vi "AnalyzeGraph.vi"(0 "Grp_Raw":waveform(dbl)[](graph), 5 "start samples/time":dbl caption="시작 샘플/시간" format="%0.2f", 7 "FittingPara":T1={"HorL_Threshold"=0.0, "HorR_Threshold"=0.0, "HorPk Width"=2, "VerL_Threshold"=0.0, "VerR_Threshold"=0.0, "VerPk Width"=2, "TorL_Threshold 3"=0.0, "TorR_Threshold"=0.0, "TorPk Width 3"=2}, 9 "duration":dbl=1.0 caption="지속기간" format="%0.2f") -> (3 "Grp_ExtVel":waveform(dbl)[](graph), 4 "Grp_ExtPos":waveform(dbl)[](graph), 6 "Hor_CycleOut":waveform(dbl)[](array[waveform]), 8 "Table_Out":dbl[][](array[numeric]), 10 "HV_CycleOut":waveform(dbl)(graph), 11 "Basic_Detection":cluster{"period":dbl, "mean":dbl, dbl}, 12 "Ver_CycleOut":waveform(dbl)[](array[waveform]), 13 "SNTable_Out":dbl[][](array[numeric]), 14 "Grph_Dir":bool, 15 "Tor_CycleOut":waveform(dbl)[](array[waveform]))   [LabVIEW 2013]
uses:
  <vilib>/Analysis/baseanly.llb/Mean (DBL).vi
  <vilib>/Waveform/WDTOps.llb/WDT Get Waveform Subset DBL.vi
  <vilib>/Waveform/WDTOps.llb/WDT Waveform Duration DBL.vi
  <vilib>/measure/mascope.llb/Pulse Measurements 1 chan.vi
  <vilib>/addons/Wavelet Analysis/application.llb/WA Multiscale Peak Detection (Waveform).vi
  <vilib>/measure/NI_MAPro.lvlib
  <vilib>/Analysis/NI_AAL_SigProc.lvlib
  <vilib>/Analysis/NI_AALBase.lvlib
  <vilib>/addons/_Advanced Signal Processing/NI_AdvSigProcWA.lvlib
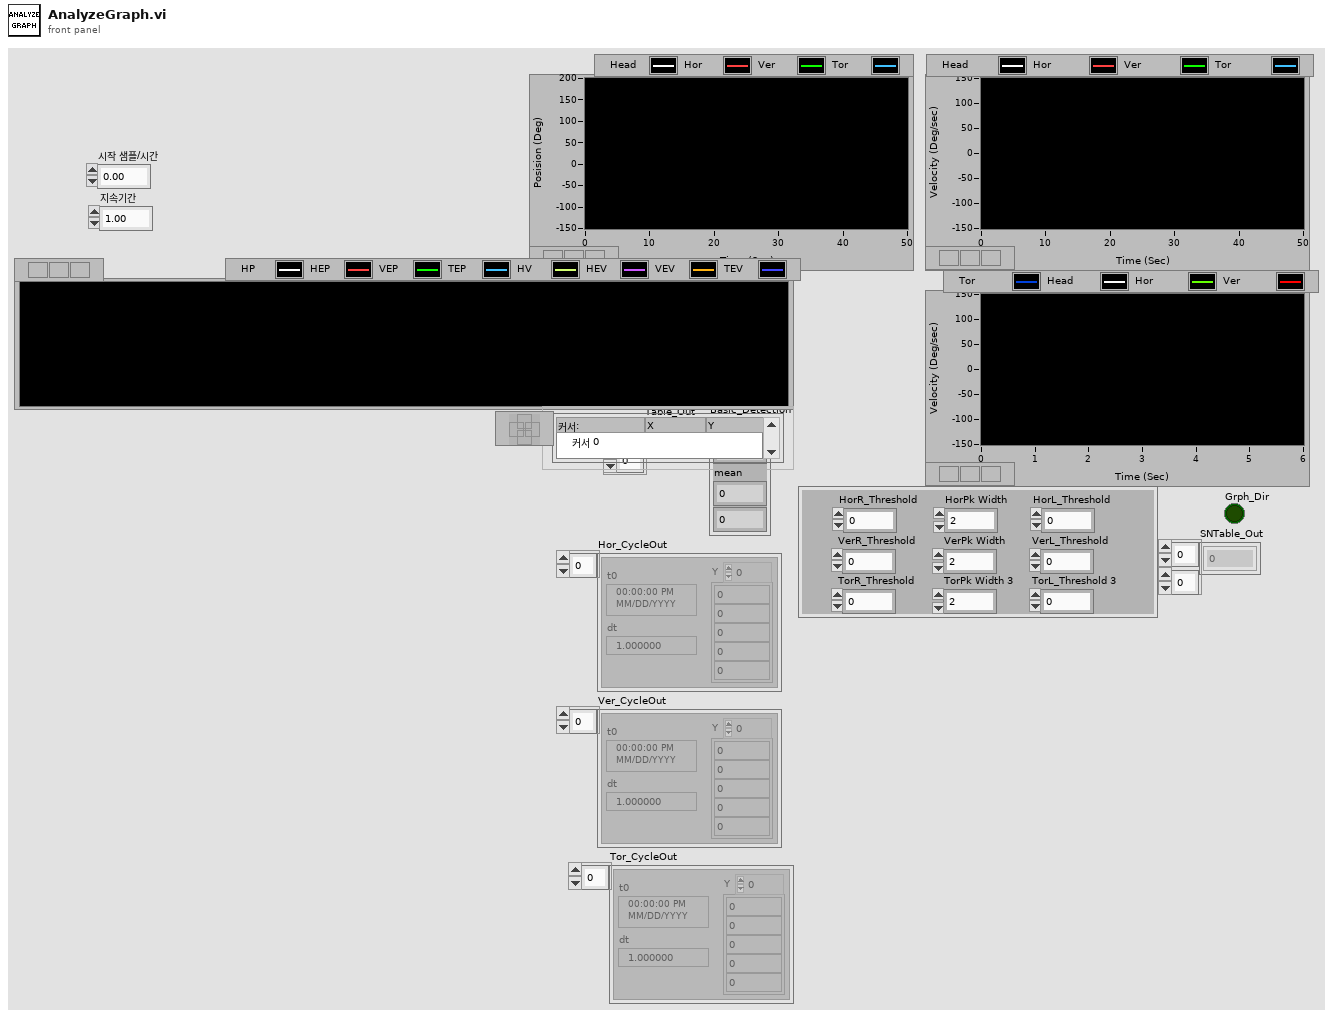
[diagram p1: front panel]
types:
  T1 = cluster{"HorL_Threshold":dbl, "HorR_Threshold":dbl, "HorPk Width":i32, "VerL_Threshold":dbl, "VerR_Threshold":dbl, "VerPk Width":i32, "TorL_Threshold 3":dbl, "TorR_Threshold":dbl, "TorPk Width 3":i32}
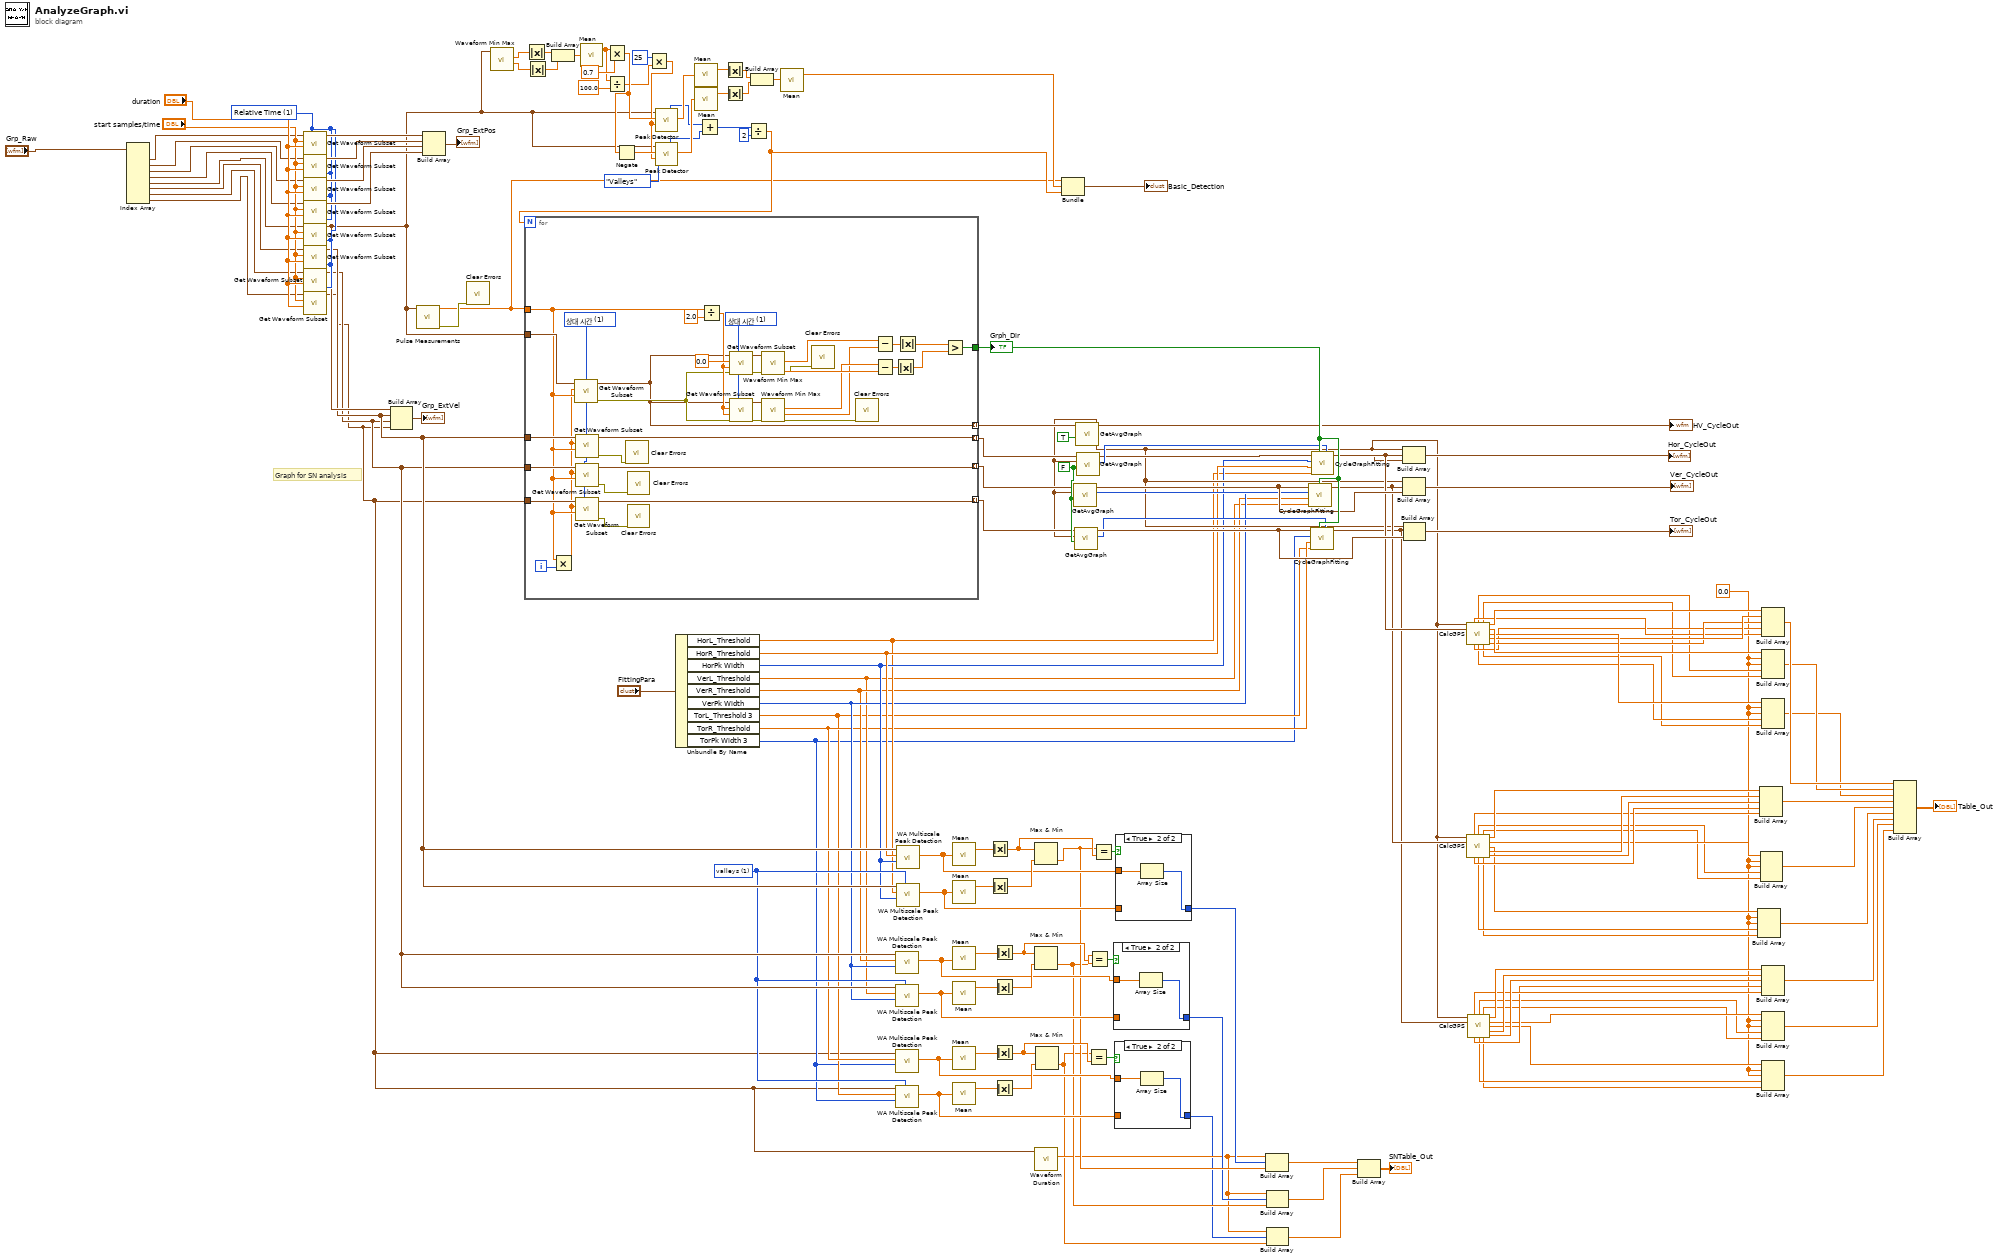
[diagram p0: block diagram]
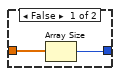
[diagram p2: hidden frame]
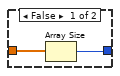
[diagram p3: hidden frame]
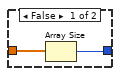
[diagram p4: hidden frame]
diagram:
  w43 = u16 1 items=["peaks", "valleys"] ("peaks/valleys")
  w48 = 0.0 ("element")
  w110 = FALSE ("HV?")
  w113 = u16 1 items=["Samples", "Relative Time"] ("start/duration format")
  # "Graph for SN analysis"
  n1 = Index Array(array="Grp_Raw") -> (element #1=w122:waveform(dbl), element #2=w121:waveform(dbl), element #3=w120:waveform(dbl), element #4=w119:waveform(dbl), element #5=w118:waveform(dbl), element #6=w117:waveform(dbl), element #7=w116:waveform(dbl), element #8=w115:waveform(dbl))  [unwired: 8 in]
  n2 = call-poly <vilib>:"Get Waveform Subset.vi"("start/duration format"=w113, "duration"="duration", "start samples/time"="start samples/time", "waveform in"=w122) -> ("waveform out"=w128:waveform(dbl))  [unwired: 2 in, 3 out]
  n3 = call-poly <vilib>:"Get Waveform Subset.vi"("start/duration format"=w113, "duration"="duration", "start samples/time"="start samples/time", "waveform in"=w121) -> ("waveform out"=w127:waveform(dbl))  [unwired: 2 in, 3 out]
  n4 = call-poly <vilib>:"Get Waveform Subset.vi"("start/duration format"=w113, "duration"="duration", "start samples/time"="start samples/time", "waveform in"=w120) -> ("waveform out"=w126:waveform(dbl))  [unwired: 2 in, 3 out]
  n5 = call-poly <vilib>:"Get Waveform Subset.vi"("start/duration format"=w113, "duration"="duration", "start samples/time"="start samples/time", "waveform in"=w119) -> ("waveform out"=w125:waveform(dbl))  [unwired: 2 in, 3 out]
  n6 = call-poly <vilib>:"Get Waveform Subset.vi"("start/duration format"=w113, "duration"="duration", "start samples/time"="start samples/time", "waveform in"=w118) -> ("waveform out"=w112:waveform(dbl))  [unwired: 2 in, 3 out]
  n7 = call-poly <vilib>:"Get Waveform Subset.vi"("start/duration format"=w113, "duration"="duration", "start samples/time"="start samples/time", "waveform in"=w117) -> ("waveform out"=w45:waveform(dbl))  [unwired: 2 in, 3 out]
  n8 = call-poly <vilib>:"Get Waveform Subset.vi"("start/duration format"=w113, "duration"="duration", "start samples/time"="start samples/time", "waveform in"=w116) -> ("waveform out"=w44:waveform(dbl))  [unwired: 2 in, 3 out]
  n9 = call-poly <vilib>:"Get Waveform Subset.vi"("start/duration format"=w113, "duration"="duration", "start samples/time"="start samples/time", "waveform in"=w115) -> ("waveform out"=w24:waveform(dbl))  [unwired: 2 in, 3 out]
  n10 = Build Array(w112, w45, w44, w24) -> (→"Grp_ExtVel":waveform(dbl)[])
  n11 = call-poly <vilib>:"Pulse Measurements.vi"("signal in"=w112) -> ("error out"=w147:errorcluster, "period"=w93:dbl)  [unwired: 6 in, 3 out]
  n12 = Build Array(w128, w127, w126, w125) -> (→"Grp_ExtPos":waveform(dbl)[])
  n13 = call <vilib>:"Clear Errors.vi"("error in (no error)"=w147) -> ()  [unwired: 6 in, 1 out]
  n14 = call <vilib>:"Waveform Min Max.vi"("waveform in"=w112) -> ("Y min"=w143:dbl, "Y max"=w144:dbl)  [unwired: 5 in, 4 out]
  n15 = Absolute Value(x=w144) -> (abs(x)=w142:dbl)
  n16 = Absolute Value(x=w143) -> (abs(x)=w141:dbl)
  n17 = Build Array(w142, w141) -> (w140:dbl[])
  n18 = call-poly <vilib>:"Mean.vi"("X"=w140) -> ("mean"=w135:dbl)  [unwired: 1 out]
  n19 = Multiply(x=w135, y=0.7) -> (x*y=w137:dbl)
  n20 = Divide(x=w135, y=100.0) -> (x/y=w133:dbl)
  n21 = Negate(x=w137) -> (-x=w138:dbl)
  n22 = Multiply(x=25 ("width"), y=w133) -> (x*y=w132:dbl)
  n23 = call <vilib>:"Peak Detector.vi"("width"=w132, "threshold"=w137, "X"=w112) -> ("Amplitudes"=w158:dbl[], "# found"=w154:i32)  [unwired: 4 in, 3 out]
  n24 = call <vilib>:"Peak Detector.vi"("peaks/valleys"=enum32{"Peaks", "Valleys"}."Valleys", "width"=w132, "threshold"=w138, "X"=w112) -> ("Amplitudes"=w157:dbl[], "# found"=w153:i32)  [unwired: 3 in, 3 out]
  n25 = Unbundle By Name("FittingPara") -> ("HorL_Threshold"=w31:dbl, "HorR_Threshold"=w33:dbl, "HorPk Width"=w32:i32, "VerL_Threshold"=w28:dbl, "VerR_Threshold"=w29:dbl, "VerPk Width"=w30:i32, "TorL_Threshold 3"=w26:dbl, "TorR_Threshold"=w27:dbl, "TorPk Width 3"=w25:i32)
  n26 = call-poly <vilib>:"Mean.vi"("X"=w158) -> ("mean"=w152:dbl)  [unwired: 1 out]
  n27 = call-poly <vilib>:"Mean.vi"("X"=w157) -> ("mean"=w151:dbl)  [unwired: 1 out]
  n28 = Add(x=w154, y=w153) -> (x+y=w156:i32)
  n29 = Absolute Value(x=w152) -> (abs(x)=w150:dbl)
  n30 = Absolute Value(x=w151) -> (abs(x)=w149:dbl)
  n31 = Divide(x=w156, y=2) -> (x/y=w129:dbl)
  n32 = for {
    N: w129 -> [_]
    tunnel: w93 -> [w170]
    tunnel: w112 -> [w194]
    tunnel: w45 -> [w173]
    tunnel: w44 -> [w172]
    tunnel: w24 -> [w171]
    tunnel: [w168] -> w108 mode=indexing
    tunnel: [w167] -> w107 mode=indexing
    tunnel: [w166] -> w106 mode=indexing
    tunnel: [w164] -> w91
    tunnel: [w163] -> w109 mode=indexing
    i -> [w193]
    w186 = u16 1 items=["샘플 ", "상대 시간"] ("start/duration format")
    w165 = u16 1 items=["샘플 ", "상대 시간"] ("start/duration format")
    n33 = Multiply(x=w170, y=w193) -> (x*y=w169:dbl)
    n34 = call-poly <vilib>:"Get Waveform Subset.vi"("start/duration format"=w165, "duration"=w170, "start samples/time"=w169, "waveform in"=w194) -> ("error out"=w179:errorcluster, "waveform out"=w163:waveform(dbl))  [unwired: 2 in, 2 out]
    n35 = call-poly <vilib>:"Get Waveform Subset.vi"("start/duration format"=w165, "duration"=w170, "start samples/time"=w169, "waveform in"=w173) -> ("error out"=w162:errorcluster, "waveform out"=w168:waveform(dbl))  [unwired: 2 in, 2 out]
    n36 = call-poly <vilib>:"Get Waveform Subset.vi"("start/duration format"=w165, "duration"=w170, "start samples/time"=w169, "waveform in"=w172) -> ("error out"=w161:errorcluster, "waveform out"=w167:waveform(dbl))  [unwired: 2 in, 2 out]
    n37 = call-poly <vilib>:"Get Waveform Subset.vi"("start/duration format"=w165, "duration"=w170, "start samples/time"=w169, "waveform in"=w171) -> ("error out"=w160:errorcluster, "waveform out"=w166:waveform(dbl))  [unwired: 2 in, 2 out]
    n38 = call <vilib>:"Clear Errors.vi"("error in (no error)"=w162) -> ()  [unwired: 6 in, 1 out]
    n39 = call <vilib>:"Clear Errors.vi"("error in (no error)"=w161) -> ()  [unwired: 6 in, 1 out]
    n40 = call <vilib>:"Clear Errors.vi"("error in (no error)"=w160) -> ()  [unwired: 6 in, 1 out]
    n41 = Divide(x=w170, y=2.0) -> (x/y=w187:dbl)
    n42 = call-poly <vilib>:"Get Waveform Subset.vi"("start/duration format"=w186, "error in (no error)"=w179, "duration"=w187, "start samples/time"=0.0, "waveform in"=w163) -> ("error out"=w181:errorcluster, "waveform out"=w191:waveform(dbl))  [unwired: 1 in, 2 out]
    n43 = call-poly <vilib>:"Get Waveform Subset.vi"("start/duration format"=w186, "error in (no error)"=w179, "duration"=w187, "start samples/time"=w187, "waveform in"=w163) -> ("error out"=w180:errorcluster, "waveform out"=w190:waveform(dbl))  [unwired: 1 in, 2 out]
    n44 = call <vilib>:"Waveform Min Max.vi"("error in (no error)"=w181, "waveform in"=w191) -> ("error out"=w178:errorcluster, "Y min"=w189:dbl, "Y max"=w176:dbl)  [unwired: 4 in, 3 out]
    n45 = call <vilib>:"Waveform Min Max.vi"("error in (no error)"=w180, "waveform in"=w190) -> ("error out"=w177:errorcluster, "Y min"=w174:dbl, "Y max"=w175:dbl)  [unwired: 4 in, 3 out]
    n46 = call <vilib>:"Clear Errors.vi"("error in (no error)"=w178) -> ()  [unwired: 6 in, 1 out]
    n47 = call <vilib>:"Clear Errors.vi"("error in (no error)"=w177) -> ()  [unwired: 6 in, 1 out]
    n48 = Subtract(x=w176, y=w174) -> (x-y=w185:dbl)
    n49 = Subtract(x=w175, y=w189) -> (x-y=w183:dbl)
    n50 = Absolute Value(x=w183) -> (abs(x)=w182:dbl)
    n51 = Absolute Value(x=w185) -> (abs(x)=w184:dbl)
    n52 = Greater?(x=w184, y=w182) -> (0:w164:bool)
  }
  "Grph_Dir" <- w91
  n53 = Build Array(w150, w149) -> (w148:dbl[])
  n54 = call-poly <vilib>:"Mean.vi"("X"=w148) -> ("mean"=w130:dbl)  [unwired: 1 out]
  n55 = call-poly <vilib>:"WA Multiscale Peak Detection.vi"("width"=w30, "threshold"=w29, "signal"=w44) -> ("amplitude"=w17:dbl[])  [unwired: 4 in, 4 out]
  n56 = call-poly <vilib>:"WA Multiscale Peak Detection.vi"("peaks/valleys"=w43, "width"=w30, "threshold"=w28, "signal"=w44) -> ("amplitude"=w16:dbl[])  [unwired: 3 in, 4 out]
  n57 = call-poly <vilib>:"WA Multiscale Peak Detection.vi"("width"=w25, "threshold"=w27, "signal"=w24) -> ("amplitude"=w14:dbl[])  [unwired: 4 in, 4 out]
  n58 = call-poly <vilib>:"WA Multiscale Peak Detection.vi"("peaks/valleys"=w43, "width"=w25, "threshold"=w26, "signal"=w24) -> ("amplitude"=w13:dbl[])  [unwired: 3 in, 4 out]
  n59 = call-poly <vilib>:"WA Multiscale Peak Detection.vi"("width"=w32, "threshold"=w33, "signal"=w45) -> ("amplitude"=w21:dbl[])  [unwired: 4 in, 4 out]
  n60 = call-poly <vilib>:"WA Multiscale Peak Detection.vi"("peaks/valleys"=w43, "width"=w32, "threshold"=w31, "signal"=w45) -> ("amplitude"=w20:dbl[])  [unwired: 3 in, 4 out]
  n61 = call-poly <vilib>:"Mean.vi"("X"=w21) -> ("mean"=w42:dbl)  [unwired: 1 out]
  n62 = call-poly <vilib>:"Mean.vi"("X"=w20) -> ("mean"=w41:dbl)  [unwired: 1 out]
  n63 = call-poly <vilib>:"Mean.vi"("X"=w17) -> ("mean"=w39:dbl)  [unwired: 1 out]
  n64 = call-poly <vilib>:"Mean.vi"("X"=w16) -> ("mean"=w38:dbl)  [unwired: 1 out]
  n65 = call-poly <vilib>:"Mean.vi"("X"=w14) -> ("mean"=w36:dbl)  [unwired: 1 out]
  n66 = call-poly <vilib>:"Mean.vi"("X"=w13) -> ("mean"=w35:dbl)  [unwired: 1 out]
  n67 = Absolute Value(x=w42) -> (abs(x)=w22:dbl)
  n68 = Absolute Value(x=w41) -> (abs(x)=w40:dbl)
  n69 = Absolute Value(x=w39) -> (abs(x)=w18:dbl)
  n70 = Absolute Value(x=w38) -> (abs(x)=w37:dbl)
  n71 = Absolute Value(x=w36) -> (abs(x)=w15:dbl)
  n72 = Absolute Value(x=w35) -> (abs(x)=w34:dbl)
  n73 = Max & Min(x=w22, y=w40) -> (min(x,y)=w11:dbl)  [unwired: 1 out]
  n74 = Max & Min(x=w18, y=w37) -> (min(x,y)=w9:dbl)  [unwired: 1 out]
  n75 = call-poly <vilib>:"Waveform Duration.vi"("waveform in"=w24) -> ("duration"=w8:dbl)  [unwired: 8 in, 2 out]
  n76 = Max & Min(x=w15, y=w34) -> (min(x,y)=w6:dbl)  [unwired: 1 out]
  n77 = Bundle("period"=w93, "mean"=w130, w129) -> (→"Basic_Detection":cluster{"period":dbl, "mean":dbl, dbl})  [unwired: 1 in]
  n78 = call "GetAvgGraph.vi"("HV?"=TRUE, "Grph_In"=w109) -> ("Grph_Avg"=w47:waveform(dbl))  [unwired: 8 in, 1 out]
  "HV_CycleOut" <- w47
  n79 = call "GetAvgGraph.vi"("HV?"=w110, "HVGrph_In"=w47, "Grph_In"=w107) -> ("Numeric"=w87:i32, "Grph_Avg"=w90:waveform(dbl))  [unwired: 7 in]
  n80 = call "GetAvgGraph.vi"("HV?"=w110, "HVGrph_In"=w47, "Grph_In"=w106) -> ("Numeric"=w86:i32, "Grph_Avg"=w89:waveform(dbl))  [unwired: 7 in]
  n81 = call "GetAvgGraph.vi"("HV?"=w110, "HVGrph_In"=w47, "Grph_In"=w108) -> ("Numeric"=w88:i32, "Grph_Avg"=w82:waveform(dbl))  [unwired: 7 in]
  n82 = Equal?(x=w6, y=w15) -> (x = y?=w1:bool)
  n83 = Equal?(x=w9, y=w18) -> (x = y?=w19:bool)
  n84 = Equal?(x=w11, y=w22) -> (x = y?=w23:bool)
  n85 = case shown="True" w19 {
    tunnel: w17 -> [_ w198]
    tunnel: w16 -> [w196 _]
    tunnel: [w195 w197] -> w10
    frame False {
      n86 = Array Size(array=w196) -> (size(s)=w195:i32)
    }
    frame True {
      n87 = Array Size(array=w198) -> (size(s)=w197:i32)
    }
  }
  n88 = case shown="True" w1 {
    tunnel: w14 -> [_ w202]
    tunnel: w13 -> [w200 _]
    tunnel: [w199 w201] -> w7
    frame False {
      n89 = Array Size(array=w200) -> (size(s)=w199:i32)
    }
    frame True {
      n90 = Array Size(array=w202) -> (size(s)=w201:i32)
    }
  }
  n91 = case shown="True" w23 {
    tunnel: w21 -> [_ w206]
    tunnel: w20 -> [w204 _]
    tunnel: [w203 w205] -> w12
    frame False {
      n92 = Array Size(array=w204) -> (size(s)=w203:i32)
    }
    frame True {
      n93 = Array Size(array=w206) -> (size(s)=w205:i32)
    }
  }
  n94 = Build Array(w8, w12, w11) -> (w5:dbl[])
  n95 = Build Array(w8, w10, w9) -> (w4:dbl[])
  n96 = Build Array(w8, w7, w6) -> (w3:dbl[])
  n97 = call "CycleGraphFitting.vi"("samples"=w87, "Grph_Dir"=w91, "L_Threshold"=w28, "R_Threshold"=w29, "width"=w30, "signal"=w90) -> ("출력 웨이브폼"=w84:waveform(dbl))  [unwired: 4 in, 1 out]
  n98 = call "CycleGraphFitting.vi"("samples"=w86, "Grph_Dir"=w91, "L_Threshold"=w26, "R_Threshold"=w27, "width"=w25, "signal"=w89) -> ("출력 웨이브폼"=w83:waveform(dbl))  [unwired: 4 in, 1 out]
  n99 = call "CycleGraphFitting.vi"("samples"=w88, "Grph_Dir"=w91, "L_Threshold"=w31, "R_Threshold"=w33, "width"=w32, "signal"=w82) -> ("출력 웨이브폼"=w85:waveform(dbl))  [unwired: 4 in, 1 out]
  n100 = Build Array(w5, w4, w3) -> (→"SNTable_Out":dbl[][])
  n101 = Build Array(w47, w85, w82) -> (→"Hor_CycleOut":waveform(dbl)[])
  n102 = Build Array(w47, w84, w90) -> (→"Ver_CycleOut":waveform(dbl)[])
  n103 = Build Array(w47, w83, w89) -> (→"Tor_CycleOut":waveform(dbl)[])
  n104 = call "CalcGPS.vi"("Grph_Stimul"=w47, "Grph_Res"=w85) -> ("AHV"=w76:dbl, "RSPV"=w74:dbl, "RHV"=w73:dbl, "AGain"=w81:dbl, "RGain"=w80:dbl, "LGain"=w79:dbl, "Phase"=w78:dbl, "ASPV"=w75:dbl, "LSPV"=w72:dbl, "LHV"=w71:dbl, "Symmetry"=w77:dbl)  [unwired: 3 in]
  n105 = call "CalcGPS.vi"("Grph_Stimul"=w47, "Grph_Res"=w84) -> ("AHV"=w66:dbl, "RSPV"=w64:dbl, "RHV"=w63:dbl, "AGain"=w70:dbl, "RGain"=w65:dbl, "LGain"=w62:dbl, "Phase"=w69:dbl, "ASPV"=w67:dbl, "LSPV"=w61:dbl, "LHV"=w60:dbl, "Symmetry"=w68:dbl)  [unwired: 3 in]
  n106 = call "CalcGPS.vi"("Grph_Stimul"=w47, "Grph_Res"=w83) -> ("AHV"=w56:dbl, "RSPV"=w53:dbl, "RHV"=w52:dbl, "AGain"=w59:dbl, "RGain"=w54:dbl, "LGain"=w51:dbl, "Phase"=w58:dbl, "ASPV"=w55:dbl, "LSPV"=w50:dbl, "LHV"=w49:dbl, "Symmetry"=w57:dbl)  [unwired: 3 in]
  n107 = Build Array(w62, w48, w48, w61, w60) -> (w97:dbl[])
  n108 = Build Array(w70, w69, w68, w67, w66) -> (w99:dbl[])
  n109 = Build Array(w65, w48, w48, w64, w63) -> (w98:dbl[])
  n110 = Build Array(w81, w78, w77, w75, w76) -> (w102:dbl[])
  n111 = Build Array(w80, w48, w48, w74, w73) -> (w101:dbl[])
  n112 = Build Array(w79, w48, w48, w72, w71) -> (w100:dbl[])
  n113 = Build Array(w59, w58, w57, w55, w56) -> (w96:dbl[])
  n114 = Build Array(w54, w48, w48, w53, w52) -> (w95:dbl[])
  n115 = Build Array(w51, w48, w48, w50, w49) -> (w94:dbl[])
  n116 = Build Array(w102, w101, w100, w99, w98, w97, w96, w95, w94) -> (→"Table_Out":dbl[][])
